vi "jog motor.vi"(8 "error in (no error)":errorcluster, 10 "CCW? (T)":bool=TRUE, 11 "Stepper in":refnum<class "Stepper.lvclass">) -> (0 "error out":errorcluster, 3 "Stepper out":refnum<class "Stepper.lvclass">)   [LabVIEW 2025, in "Stepper.lvclass"]
uses:
  Stepper.lvclass
  Stepper.lvclass/Stepper.ctl
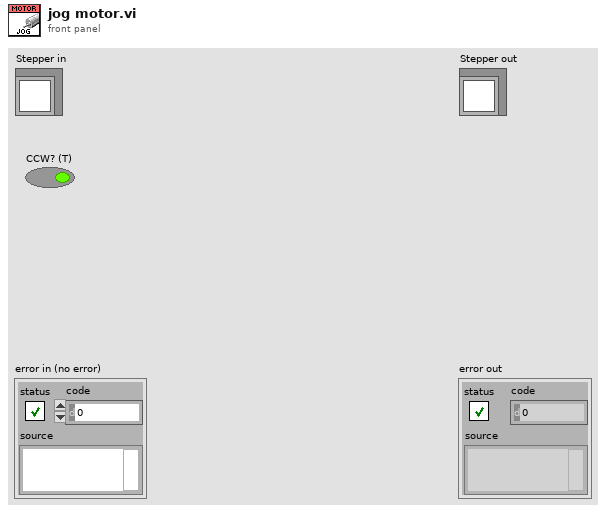
[diagram p1: front panel]
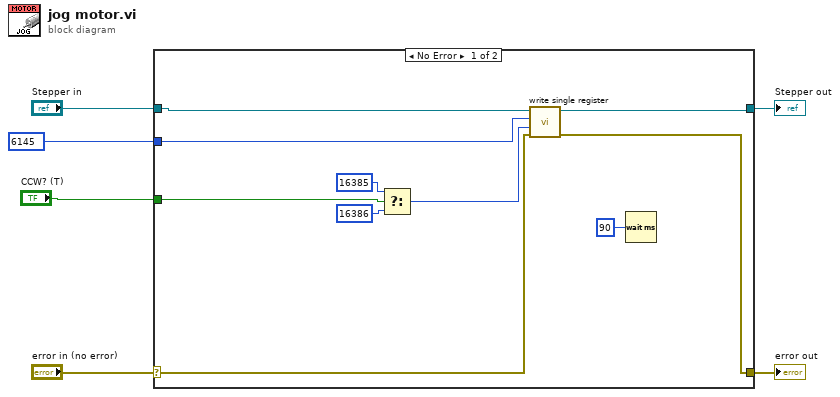
[diagram p0: block diagram]
diagram:
  n1 = case shown="No Error" "error in (no error)" {
    selector: "error in (no error)" -> [w13 w18]
    tunnel: [w14 w18] -> w5
    tunnel: [w15 w17] -> w3
    tunnel: "Stepper in" -> [w16 w17]
    tunnel: u16 6145 ("address") -> [w12 _]
    tunnel: "CCW? (T)" -> [w8 _]
    frame No Error {
      n2 = Select(t=u16 16385 ("address"), s=w8, f=u16 16386 ("address")) -> (s? t:f=w9:u16)
      n3 = call-dynamic "write single register.vi"("error in (no error)"=w13, "register to write"=w9, "address"=w12, "Stepper in"=w16) -> ("error out"=w14:errorcluster, "Stepper out"=w15:refnum<class "Stepper.lvclass">)  [unwired: 6 in]
      n4 = Wait (ms)(milliseconds to wait=u32 90) -> ()  [unwired: 1 out]
    }
    frame Error {
    }
  }
  "error out" <- w5
  "Stepper out" <- w3
